vi "SA_GotoPositionAbsolute_S.vi"(5 "channelIndex":u32, 7 "systemIndex":u32, 8 "error in (no error)":errorcluster, 10 "holdTime":u32 max=60000, 11 "position":i32) -> (0 "error out":errorcluster)   [LabVIEW 2013]
doc: "<B>Description:</B>\nInstructs a positioner to move to a specific position. This function is only executable by a positioner that has a sensor attached to it. The sensor must also be enabled or in power save mode (see SA_SetSensorEnabled_S). If this is not the case an error will be returned. Additionally, the command is only executable if the addressed channel is configured to be of type linear (see SA_SetSensorType_S). A rotary channel will return an error. See also SA_GotoAngleAbsolute_S.\nThe positioner may be instructed to hold the target position after it has been reached. This may be useful to compensate for drift effects and the like. Note that the positioner will use the scan mode to hold the position if needed. When the piezo element of the positioner reaches a scanning boundary a single step is performed. However, if this behavior is not desired the correction steps can be disabled with the SA_SetStepWhileScan_S command (see there). Note though that disabling the steps might mean that the position cannot be held.\nWhile executing the command the positioner will have a movement status of SA_TARGET_STATUS. While holding the target position the positioner will have a movement status of SA_HOLDING_STATUS (see SA_GetStatus_S).\nIf a mechanical end stop is detected while the command is in execution, the movement will be aborted. Note that in asynchronous communication mode an error will be reported.\n<B>Parameters:</B>\n<B>- systemIndex</B> (unsigned 32bit), input - Selects the system. The index is zero based.\n<B>- channelIndex</B> (unsigned 32bit), input - Selects the channel of the selected system. The index is zero based.\n<B>- position</B> (signed 32bit), input - Absolute position to move to in nano meters.\n<B>- holdTime</B> (unsigned 32bit), input - Specifies how long (in milliseconds) the position is actively held after reaching the target. The valid range is 0..60,000. A 0 deactivates this feature, a value of 60,000 is infinite (until manually stopped, see SA_Stop_S)."
uses:
  MCSControl.dll
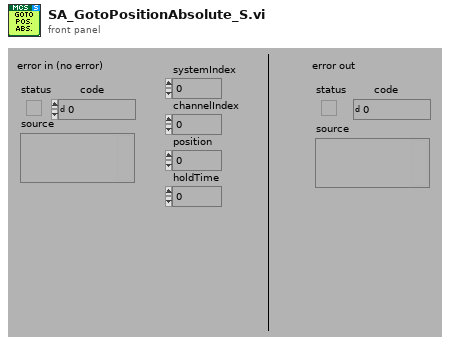
[diagram p1: front panel]
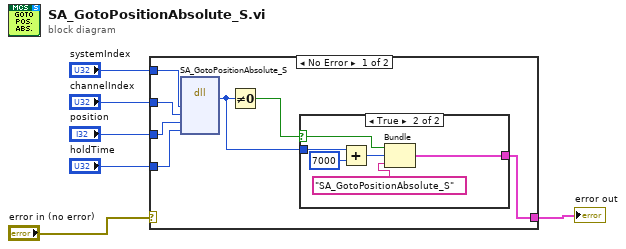
[diagram p0: block diagram]
diagram:
  n1 = case shown="No Error" "error in (no error)" {
    selector: "error in (no error)" -> [_ w20]
    tunnel: [w11 w20] -> w5
    tunnel: "systemIndex" -> [w10 _]
    tunnel: "channelIndex" -> [w9 _]
    tunnel: "position" -> [w8 _]
    tunnel: "holdTime" -> [w7 _]
    frame No Error {
      n2 = dll-call lib="MCSControl.dll" fn="SA_GotoPositionAbsolute_S"("systemIndex"=w10, "channelIndex"=w9, "position"=w8, "holdTime"=w7) -> (w12:u32)  [unwired: 7 in, 2 out]
      n3 = Not Equal To 0?(x=w12) -> (x != 0?=w13:bool)
      n4 = case shown="True" w13 {
        selector: w13 -> [_ w16]
        tunnel: w12 -> [_ w19]
        tunnel: [_ w14] -> w11
        frame False {
        }
        frame True {
          n5 = Add(x=w19, y=u32 7000) -> (x+y=w17:u32)
          n6 = Bundle(w16, w17, "source"="SA_GotoPositionAbsolute_S") -> (w14:cluster{bool, u32, "source":string})  [unwired: 1 in]
        }
      }
    }
    frame Error {
    }
  }
  "error out" <- w5
